vi "sub_vi_calibration.vi"(8 "error in (no error)":errorcluster, 10 "Gain":u16, 11 "VISA resource name":refnum<visa-resource-name>) -> (0 "error out":errorcluster, 1 "Weights":dbl[](array[numeric]), 2 "Measures":dbl[](array[numeric]), 3 "VISA resource name out":refnum<visa-resource-name>)   [LabVIEW 2019]
uses:
  <vilib>/Analysis/baseanly.llb/Mean (DBL).vi
  <vilib>/Analysis/NI_AALBase.lvlib
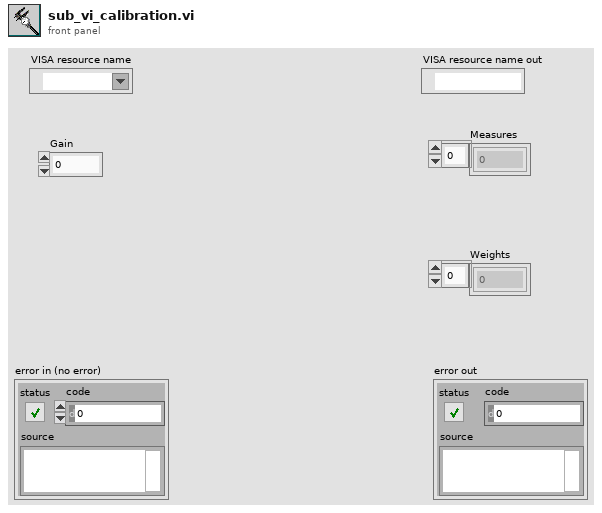
[diagram p1: front panel]
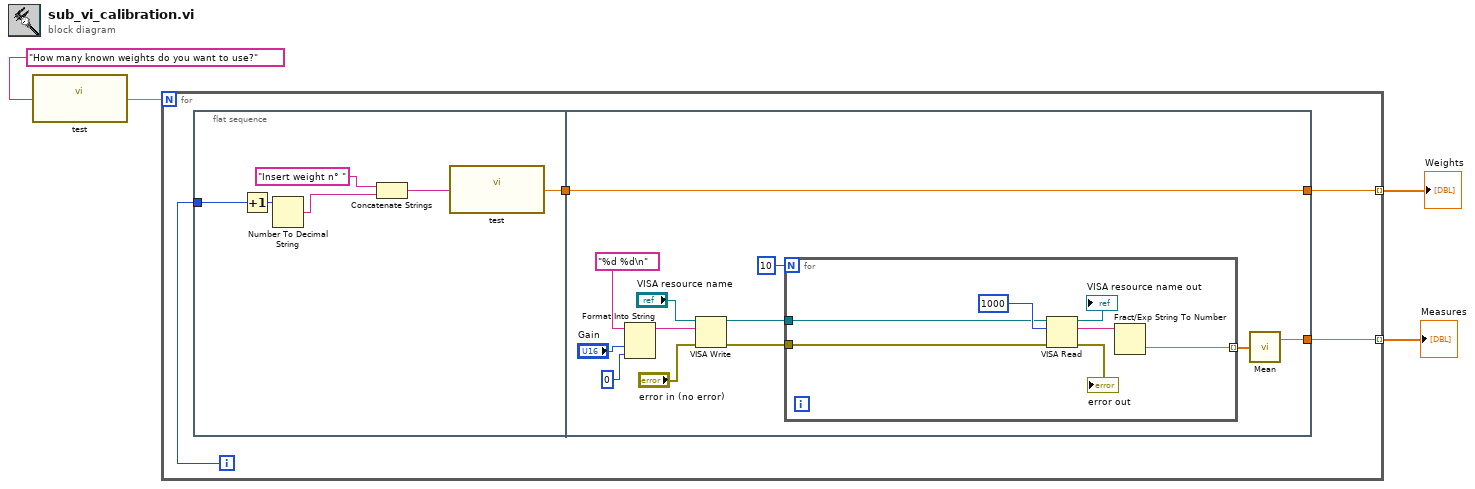
[diagram p0: block diagram]
diagram:
  n1 = call "test.vi"("Title"="How many known weights do you want to use?") -> ("Weights number 2"=w2:dbl)  [unwired: 18 in]
  n2 = for {
    N: w2 -> [_]
    tunnel: [w7] -> w3 mode=indexing
    tunnel: [w5] -> w1 mode=indexing
    i -> [w8]
    n3 = flat-sequence {
      tunnel: w8 -> [w11]
      tunnel: [w9] -> w6
      tunnel: [w26] -> w7
      tunnel: w6 -> [w26]
      tunnel: [w15] -> w5
      frame #0 {
        n4 = Increment(x=w11) -> (x+1=w14:i32)
        n5 = Number To Decimal String(number=w14) -> (decimal integer string=w13:string)  [unwired: 1 in]
        n6 = Concatenate Strings("Insert weight n° ", w13) -> (w12:string)
        n7 = call "test.vi"("Title"=w12) -> ("Weights number 2"=w9:dbl)  [unwired: 18 in]
      }
      frame #1 {
        n8 = Format Into String(format string="%d %d\n", "Gain", u16 0 ("input 2")) -> (resulting string=w22:string)  [unwired: 2 in, 1 out]
        n9 = VISA Write(VISA resource name="VISA resource name", write buffer=w22, error in (no error)="error in (no error)") -> (VISA resource name out=w18:refnum<visa-resource-name>, error out=w19:errorcluster)  [unwired: 1 out]
        n10 = for {
          N: 10 -> [_]
          tunnel: w19 -> [w29]
          tunnel: [w28] -> w16 mode=indexing
          tunnel: w18 -> [w27]
          n11 = VISA Read(VISA resource name=w27, byte count=u32 1000, error in (no error)=w29) -> (VISA resource name out=→"VISA resource name out":refnum<visa-resource-name>, read buffer=w32:string, error out=→"error out":errorcluster)  [unwired: 1 out]
          n12 = Fract/Exp String To Number(string=w32) -> (number=w28:dbl)  [unwired: 3 in, 1 out]
        }
        n13 = call-poly <vilib>:"Mean.vi"("X"=w16) -> ("mean"=w15:dbl)  [unwired: 1 out]
      }
    }
  }
  "Weights" <- w3
  "Measures" <- w1
